vi "Sobel_Edge_Detection.vi"() -> ()   [LabVIEW 2017]
uses:
  <vilib>/Analysis/Matrix/Datatypes/RealMatrix.ctl
  <vilib>/vision/NI_Vision_Development_Module.lvlib
  <vilib>/Analysis/Matrix/NI_Matrix.lvlib
panel:
  in  "y matrix":T1=[[1.0, 1.0, 1.0], [1.0, 1.0, 1.0], [1.0, 1.0, 1.0]]
  out "Numeric 2":i32
  out "Numeric":i32
  out "Image":T2(plugin-control)
  out "error out":errorcluster
  in  "error in (no error)":errorcluster
  in  "x matrix":T1=[[1.0, 1.0, 1.0], [1.0, 1.0, 1.0], [1.0, 1.0, 1.0]]
  in  "File Path":path
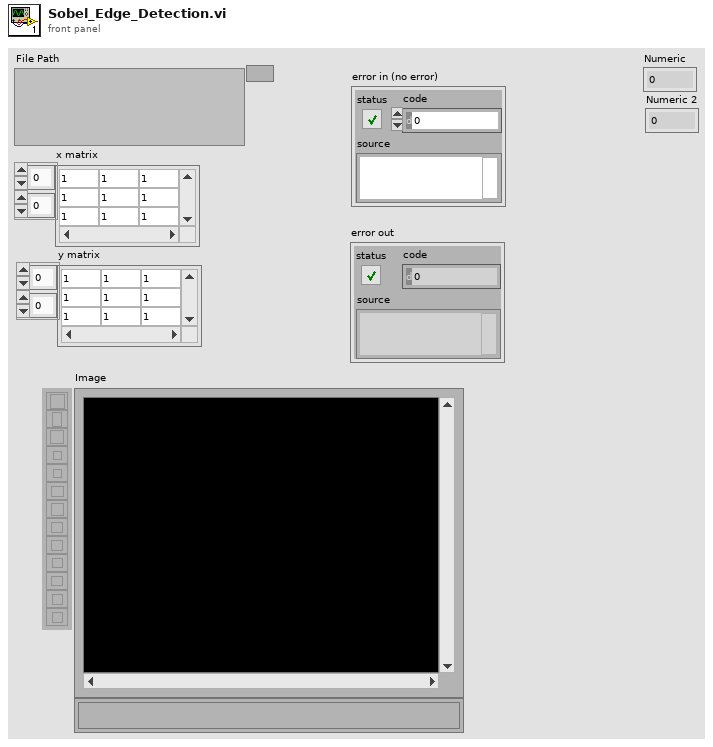
[diagram p1: front panel]
types:
  T1 = typedef "NI_Matrix.lvlib/RealMatrix.ctl" = dbl[][]
  T2 = typedef "IMAQ Image.ctl" = refnum<image>
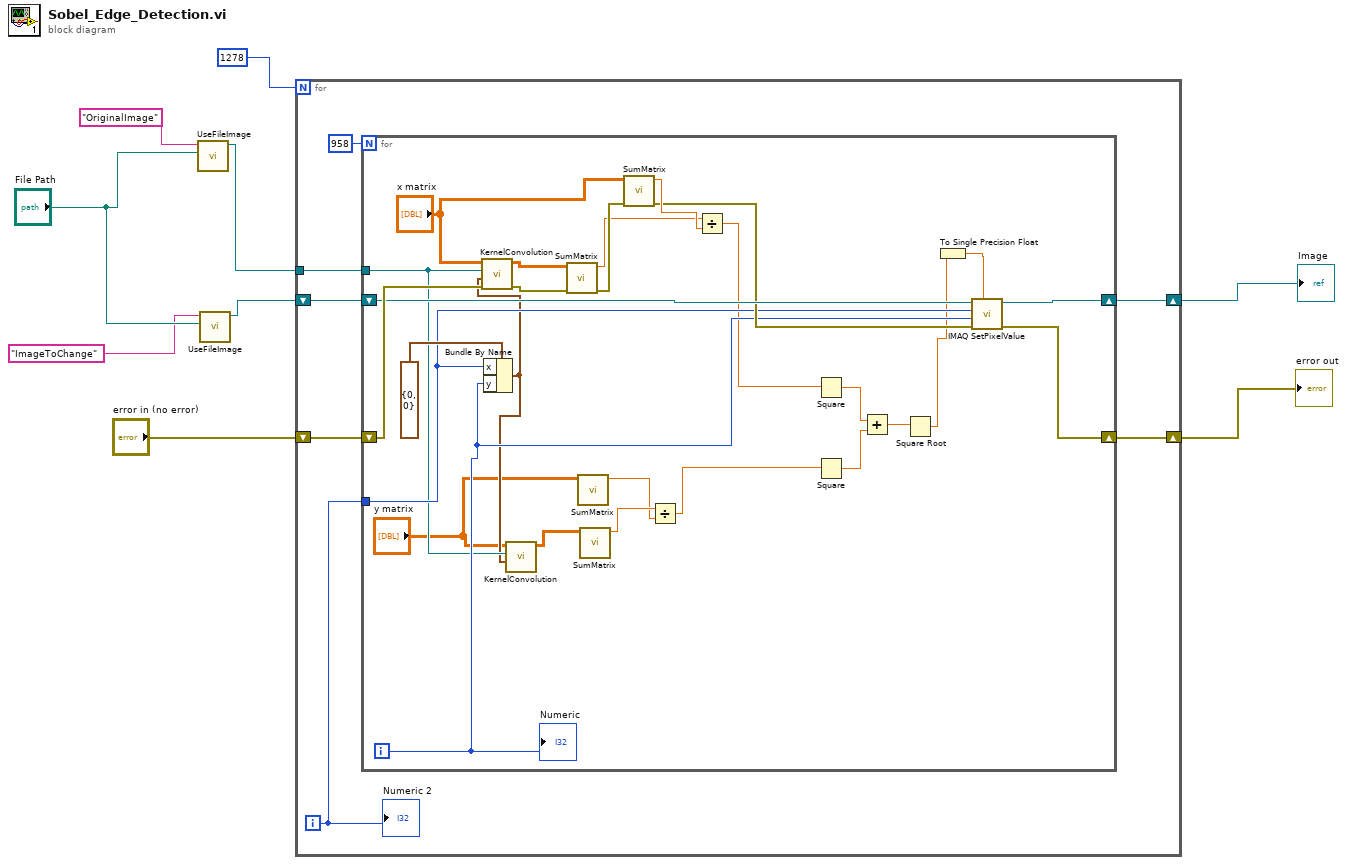
[diagram p0: block diagram]
diagram:
  n1 = call "UseFileImage.vi"("File Path"="File Path", "Image Name"="OriginalImage") -> ("Original Image"=w5:T2)  [unwired: 8 in, 1 out]
  n2 = call "UseFileImage.vi"("File Path"="File Path", "Image Name"="ImageToChange") -> ("Original Image"=w2:T2)  [unwired: 8 in, 1 out]
  n3 = for {
    N: 1278 ("Numeric") -> [_]
    tunnel: w5 -> [w15]
    shift-right: [w13] -> w3
    shift-left: "error in (no error)" -> [w14]
    shift-right: [w10] -> w1
    shift-left: w2 -> [w12]
    i -> [w11]
    n4 = for {
      N: 958 -> [_]
      tunnel: w15 -> [w28]
      shift-right: [w33] -> w13
      shift-left: w14 -> [w43]
      tunnel: w11 -> [w30]
      shift-right: [w32] -> w10
      shift-left: w12 -> [w35]
      i -> [w29]
      n5 = Bundle By Name(cluster=cluster{"x":i32, "y":i32} {"x"=0, "y"=0}, "x"=w30, "y"=w29) -> (w27:cluster{"x":i32, "y":i32})
      n6 = call "KernelConvolution.vi"("error in"=w43, "Pixel Co-ordinates"=w27, "Original Image"=w28, "matrix"="x matrix") -> ("error out"=w41:errorcluster, "NewPixelValues"=w42:T1)  [unwired: 6 in]
      n7 = call "KernelConvolution.vi"("Pixel Co-ordinates"=w27, "Original Image"=w28, "matrix"="y matrix") -> ("NewPixelValues"=w26:T1)  [unwired: 7 in, 1 out]
      n8 = call "SumMatrix.vi"("error in (no error)"=w41, "matrix"=w42) -> ("error out"=w39:errorcluster, "Sum"=w37:dbl)  [unwired: 8 in]
      n9 = call "SumMatrix.vi"("matrix"="y matrix") -> ("Sum"=w23:dbl)  [unwired: 9 in, 1 out]
      n10 = call "SumMatrix.vi"("matrix"=w26) -> ("Sum"=w24:dbl)  [unwired: 9 in, 1 out]
      n11 = call "SumMatrix.vi"("error in (no error)"=w39, "matrix"="x matrix") -> ("error out"=w34:errorcluster, "Sum"=w38:dbl)  [unwired: 8 in]
      n12 = Divide(x=w24, y=w23) -> (x/y=w22:dbl)
      n13 = Divide(x=w37, y=w38) -> (x/y=w21:dbl)
      n14 = Square(x=w21) -> (x^2=w20:dbl)
      n15 = Square(x=w22) -> (x^2=w19:dbl)
      n16 = Add(x=w20, y=w19) -> (x+y=w18:dbl)
      n17 = Square Root(x=w18) -> (sqrt(x)=w17:dbl)
      n18 = To Single Precision Float(number=w17) -> (single precision float=w36:sgl)
      n19 = call "IMAQ SetPixelValue"("Pixel Value"=w36, "error in (no error)"=w34, "Y Coordinate"=w29, "X Coordinate"=w30, "Image"=w35) -> ("error out"=w33:errorcluster, "Image Out"=w32:T2)  [unwired: 5 in]
      "Numeric" <- w29
    }
    "Numeric 2" <- w11
  }
  "error out" <- w3
  "Image" <- w1
